vi "Timer.vi"(9 "Operation":enum16{"Read", "Write"}(ring)=enum."Write", 11 "Timer Status":enum16{"Stopped", "Running"}(ring)=enum."Running") -> (0 "Sec":dbl, 1 "second":u8, 2 "Timer Status":enum16{"Stopped", "Running"}(ring), 3 "minute":u8)   [LabVIEW 2023, in "GUI.lvlib"]
uses:
  GUI.lvlib
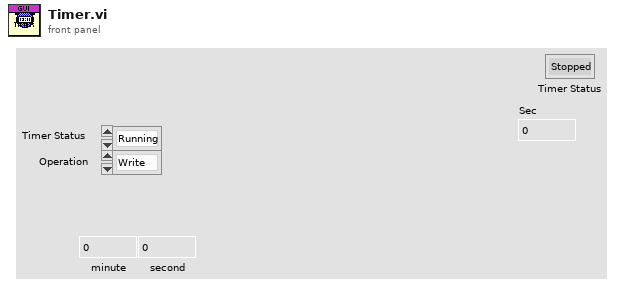
[diagram p1: front panel]
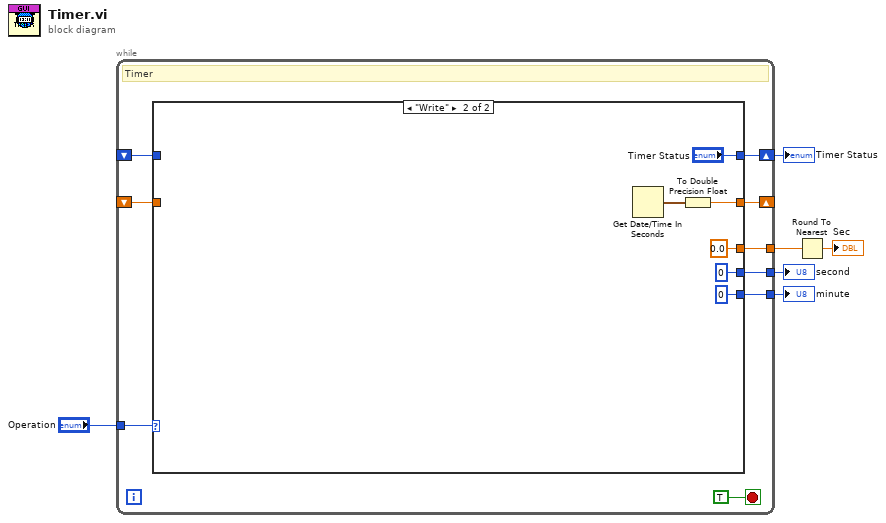
[diagram p0: block diagram]
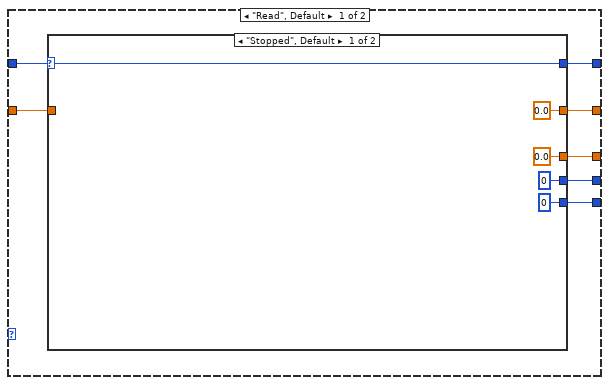
[diagram p2: hidden frame]
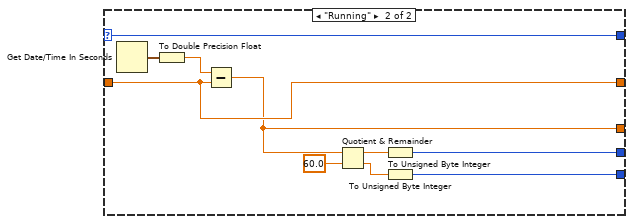
[diagram p3: hidden frame]
diagram:
  n1 = while {
    tunnel: "Operation" -> [w14]
    shift-right: [w13] -> w3
    shift-left: _ -> [w12]
    shift-right: [w11] -> _
    shift-left: _ -> [w10]
    tunnel: [w9] -> w5
    tunnel: [w8] -> w4
    tunnel: [w7] -> w2
    stop <- TRUE stop-if-true
    # "Timer"
    n2 = case shown="\"Write\"" w14 {
      tunnel: [w21 "Timer Status"] -> w13
      tunnel: w12 -> [w22 _]
      tunnel: [w19 w41] -> w11
      tunnel: w10 -> [w20 _]
      tunnel: [w18 u8 0] -> w9
      tunnel: [w17 u8 0] -> w8
      tunnel: [w16 0.0] -> w7
      frame "Read", Default {
        n3 = case shown="\"Stopped\", Default" w22 {
          selector: w22 -> [w27 w37]
          tunnel: [w27 w37] -> w21
          tunnel: w20 -> [_ w34]
          tunnel: [0.0 w34] -> w19
          tunnel: [u8 0 w30] -> w18
          tunnel: [u8 0 w29] -> w17
          tunnel: [0.0 w28] -> w16
          frame "Stopped", Default {
          }
          frame "Running" {
            n4 = Get Date/Time In Seconds() -> (seconds since 1Jan1904=w36:timestamp)
            n5 = To Double Precision Float(number=w36) -> (double precision float=w35:dbl)
            n6 = Subtract(x=w35, y=w34) -> (x-y=w28:dbl)
            n7 = Quotient & Remainder(x=w28, y=60.0) -> (x-y*floor(x/y)=w33:dbl, floor(x/y)=w32:dbl)
            n8 = To Unsigned Byte Integer(number=w33) -> (unsigned 8bit integer=w30:u8)
            n9 = To Unsigned Byte Integer(number=w32) -> (unsigned 8bit integer=w29:u8)
          }
        }
      }
      frame "Write" {
        n10 = Get Date/Time In Seconds() -> (seconds since 1Jan1904=w42:timestamp)
        n11 = To Double Precision Float(number=w42) -> (double precision float=w41:dbl)
      }
    }
  }
  "minute" <- w4
  "second" <- w5
  "Timer Status" <- w3
  n12 = Round To Nearest(number=w2) -> (nearest integer value=→"Sec":dbl)
